vi "set_message.vi"(8 "error in (no error)":errorcluster, 10 "Message":string, 11 "MoAgSy_Message.lvclass in":refnum<class "MoAgSy_Message.lvclass">) -> (0 "error out":errorcluster, 3 "MoAgSy_Message.lvclass out":refnum<class "MoAgSy_Message.lvclass">)   [LabVIEW 2009, in "MoAgSy.lvlib" / "MoAgSy_Message.lvclass"]
uses:
  MoAgSy_Message.lvclass
  MoAgSy_Message.lvclass/MoAgSy_Message.ctl
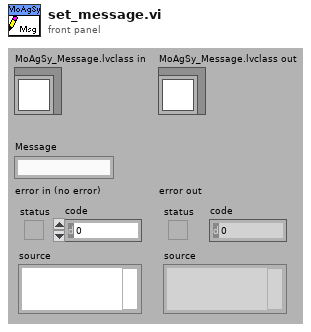
[diagram p1: front panel]
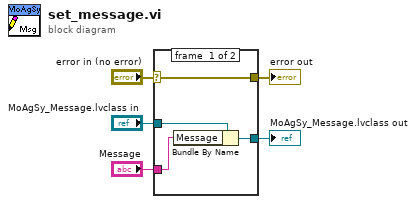
[diagram p0: block diagram]
diagram:
  n1 = case shown="No Error" "error in (no error)" {
    selector: "error in (no error)" -> [w9 w10]
    tunnel: [w9 w10] -> w4
    tunnel: [w7 w11] -> w2
    tunnel: "MoAgSy_Message.lvclass in" -> [w8 w11]
    tunnel: "Message" -> [w6 _]
    frame #0 {
      n2 = Bundle By Name(cluster=w8, "Message"=w6) -> (w7:refnum<class "MoAgSy_Message.lvclass">)
    }
    frame #1 {
    }
  }
  "error out" <- w4
  "MoAgSy_Message.lvclass out" <- w2
